vi "add timestamp to arm.vi"(11 "array of cans":T1[](array[typedef]) {"type" items=["CAN Data", "CAN Remote"]; "identifier" format="%.0x"}) -> (3 "Message Cluster":T2)   [LabVIEW 2015]
uses:
  QMH Fundamentals - Message Cluster.ctl
  RT/CANFrameControl.ctl
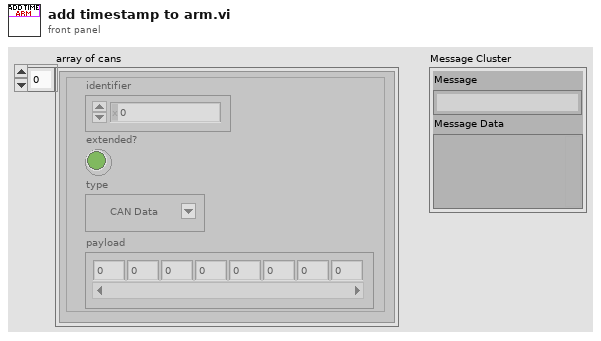
[diagram p1: front panel]
types:
  T1 = typedef "CANFrameControl.ctl" = cluster{"identifier":u32, "extended?":bool, "type":u8, "payload":u8[]}
  T2 = typedef "QMH Fundamentals - Message Cluster.ctl" = cluster{"Message":string, "Message Data":variant}
  T3 = cluster{"date/time string":string, "array of cans":T1[]}
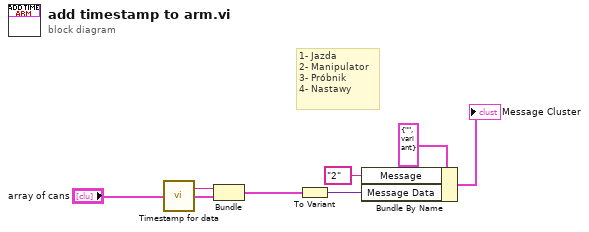
[diagram p0: block diagram]
diagram:
  # "1- Jazda\n2- Manipulator\n3- Próbnik\n4- Nastawy"
  n1 = call "Timestamp for data.vi"() -> ("date/time string"=w6:string)  [unwired: 3 in]
  n2 = Bundle("date/time string"=w6, "array of cans"="array of cans") -> (w5:T3)  [unwired: 1 in]
  n3 = To Variant(anything=w5) -> (Variant=w1:variant)
  n4 = Bundle By Name(cluster=T2 {"Message"="", "Message Data"=variant} ("Message Cluster"), "Message"="2", "Message Data"=w1) -> (→"Message Cluster":T2)
